vi "control2daq.vi"(1 "Limites":T1, 2 "Control Input":dbl[](array[numeric])) -> (0 "DAQ Output":dbl[](array[numeric]))   [LabVIEW 2010]
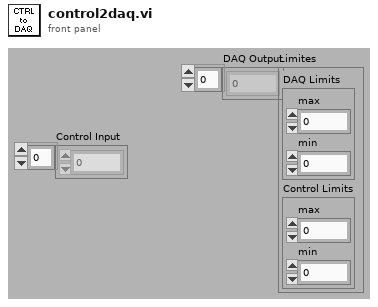
[diagram p1: front panel]
types:
  T1 = cluster{"DAQ Limits":cluster{"max":dbl, "min":dbl}, "Control Limits":cluster{"max":dbl, "min":dbl}}
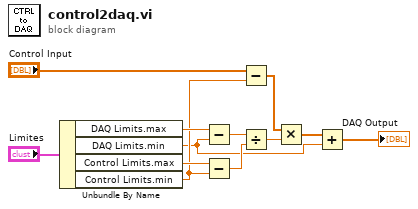
[diagram p0: block diagram]
diagram:
  n1 = Unbundle By Name("Limites") -> ("DAQ Limits.max"=w10:dbl, "DAQ Limits.min"=w3:dbl, "Control Limits.max"=w9:dbl, "Control Limits.min"=w8:dbl)
  n2 = Subtract(x=w10, y=w3) -> (x-y=w7:dbl)
  n3 = Subtract(x=w9, y=w8) -> (x-y=w6:dbl)
  n4 = Subtract(x="Control Input", y=w8) -> (x-y=w4:dbl[])
  n5 = Divide(x=w7, y=w6) -> (x/y=w5:dbl)
  n6 = Multiply(x=w4, y=w5) -> (x*y=w2:dbl[])
  n7 = Add(x=w2, y=w3) -> (x+y=→"DAQ Output":dbl[])
